vi "Database DLL Path.vi"() -> (5 "DLL Path":path)   [LabVIEW 2017]
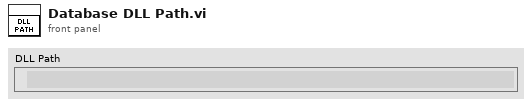
[diagram p1: front panel]
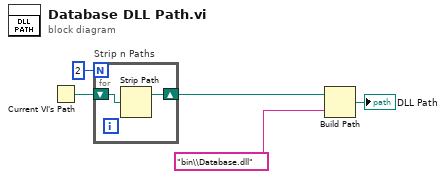
[diagram p0: block diagram]
diagram:
  n1 = Current VI's Path() -> (path=w5:path)
  n2 = for "Strip n Paths" {
    N: 2 -> [_]
    shift-right: [w6] -> w3
    shift-left: w5 -> [w7]
    n3 = Strip Path(path=w7) -> (stripped path=w6:path)  [unwired: 1 out]
  }
  n4 = Build Path(base path=w3, name or relative path="bin\\Database.dll") -> (appended path=→"DLL Path":path)
